vi "headingweightsum2.vi"(8 "a":dbl, 10 "h2":dbl, 11 "h1":dbl) -> (3 "a*h2+(1-a)*h1":dbl)   [LabVIEW 2015]
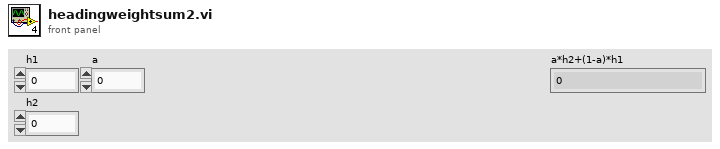
[diagram p1: front panel]
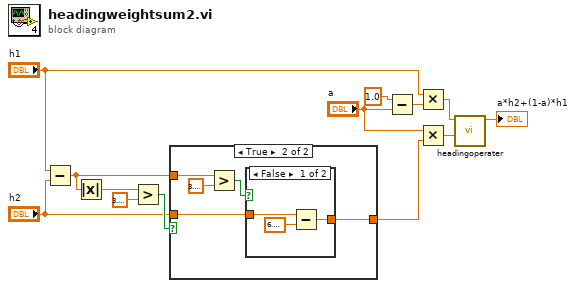
[diagram p0: block diagram]
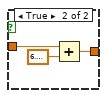
[diagram p3: hidden frame]
diagram:
  n1 = Subtract(x="h1", y="h2") -> (x-y=w10:dbl)
  n2 = Absolute Value(x=w10) -> (abs(x)=w13:dbl)
  n3 = Greater?(x=w13, y=3.141592653589793) -> (0:w11:bool)
  n4 = case shown="True" w11 {
    tunnel: w10 -> [_ w18]
    tunnel: "h2" -> [w14 w16]
    tunnel: [w14 w15] -> w8
    frame False {
    }
    frame True {
      n5 = Greater?(x=w18, y=3.141592653589793) -> (0:w17:bool)
      n6 = case shown="False" w17 {
        tunnel: w16 -> [w22 w25]
        tunnel: [w20 w23] -> w15
        frame False {
          n7 = Subtract(x=w22, y=6.283185307179586) -> (x-y=w20:dbl)
        }
        frame True {
          n8 = Add(x=w25, y=6.283185307179586) -> (x+y=w23:dbl)
        }
      }
    }
  }
  n9 = Subtract(x=1.0, y="a") -> (x-y=w1:dbl)
  n10 = Multiply(x="h1", y=w1) -> (x*y=w7:dbl)
  n11 = Multiply(x="a", y=w8) -> (x*y=w6:dbl)
  n12 = call "headingoperater.vi"("h1"=w6, "h2"=w7) -> ("h2+h1"=→"a*h2+(1-a)*h1":dbl)  [unwired: 8 in, 1 out]
